vi "LabVIEW_VTOL.vi"() -> ()   [LabVIEW 2018]
uses:
  <vilib>/Analysis/baseanly.llb/A x Vector.vi
  <vilib>/Instr/_visa.llb/VISA Configure Serial Port (Instr).vi
  <vilib>/Analysis/NI_AALBase.lvlib
panel:
  out "Yaw error integral":dbl(graph)
  out "Pitch error intergal":dbl(graph)
  in  "Yaw":dbl(slide) scale=-90.0..90.0
  in  "Pitch":dbl(slide) scale=-90.0..90.0
  out "size(s) 3":i32
  out "size(s) 2":i32
  out "Propeller 2":dbl(graph)
  out "Propeller 1":dbl(graph)
  in  "stop":bool
  out "Raw Data":string
  in  "array type (2D Dbl)":dbl[](array[numeric])
  out "Pitch":T1(graph)
  out "Roll":dbl(graph)
  out "Yaw":T1(graph)
  out "Pitch speed":dbl(graph)
  out "Roll speed":dbl(graph)
  out "Yaw speed":dbl(graph)
  in  "VISA resource name":refnum<visa-resource-name>
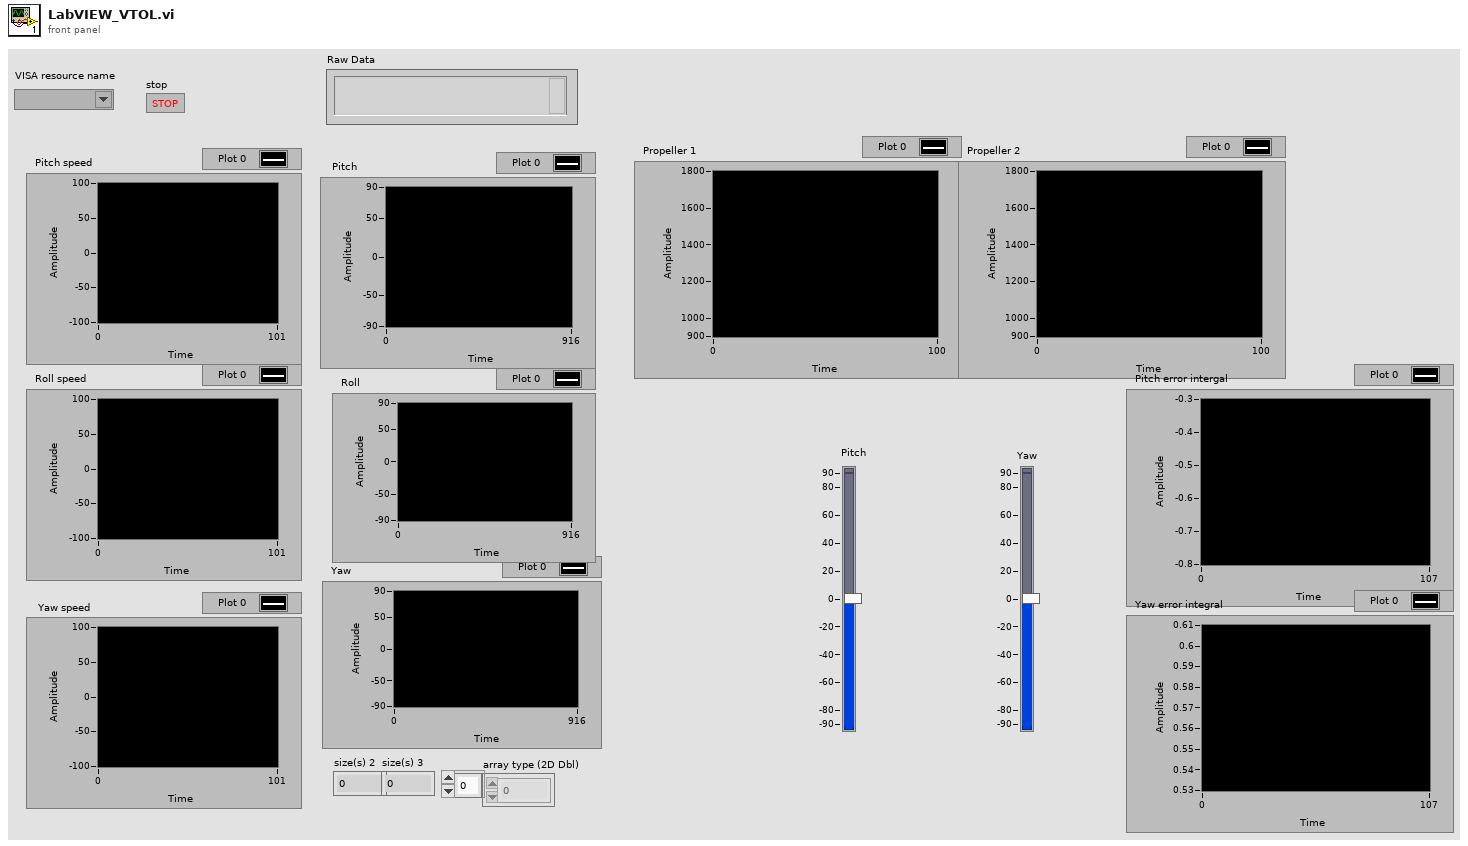
[diagram p1: front panel]
types:
  T1 = cluster{"[0]":dbl, "[1]":dbl, "[2]":dbl, "[3]":dbl, "[4]":dbl, "[5]":dbl, "[6]":dbl, "[7]":dbl, "[8]":dbl}
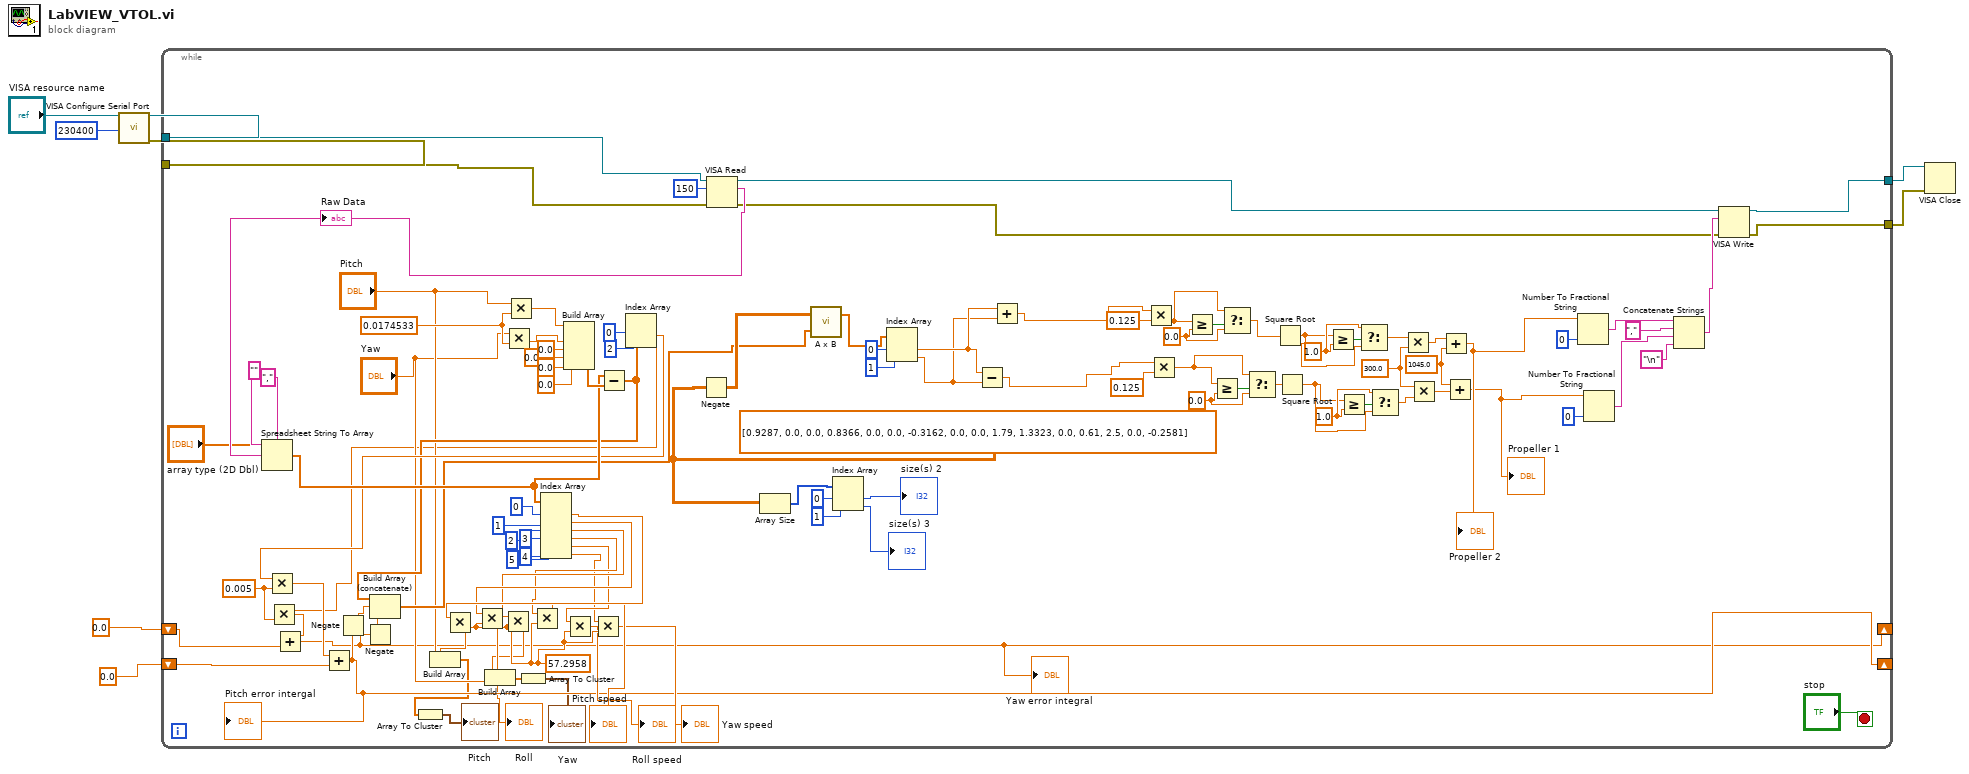
[diagram p0: block diagram]
diagram:
  n1 = call-poly "VISA Configure Serial Port"("VISA resource name"="VISA resource name", "baud rate (9600)"=u32 230400) -> ("VISA resource name out"=w7:refnum<visa-resource-name>, "error out"=w6:errorcluster)  [unwired: 12 in]
  n2 = while {
    tunnel: w7 -> [w113]
    tunnel: w6 -> [w112]
    tunnel: [w59] -> w5
    tunnel: [w56] -> w4
    shift-right: [w29] -> _
    shift-left: 0.0 -> [w14]
    shift-right: [w10] -> _
    shift-left: 0.0 -> [w12]
    stop <- "stop" stop-if-true
    w15 = 0.005 ("y")
    w41 = 0.0174533 ("y")
    w50 = 57.2958 ("y")
    w72 = 1.0 ("y")
    w76 = 1.0 ("y")
    w80 = 0.0 ("y")
    w83 = 0.0 ("y")
    w86 = 1045.0 ("y")
    w89 = 300.0 ("y")
    w9 = dbl[][] [[0.9287, 0.0, 0.0, 0.8366, 0.0, 0.0, -0.3162, 0.0], [0.0, 1.79, 1.3323, 0.0, 0.61, 2.5, 0.0, -0.2581]] ("Controller Gain")
    n3 = Multiply(x="Yaw", y=w41) -> (x*y=w31:dbl)
    n4 = Multiply(x="Pitch", y=w41) -> (x*y=w42:dbl)
    n5 = Build Array(w42, 0.0 ("element"), w31, 0.0 ("element"), 0.0 ("element"), 0.0 ("element")) -> (w37:dbl[])
    n6 = Negate(x=w9) -> (-x=w55:dbl[][])
    n7 = VISA Read(VISA resource name=w113, byte count=u32 150, error in (no error)=w112) -> (VISA resource name out=w58:refnum<visa-resource-name>, read buffer=w110:string, error out=w57:errorcluster)  [unwired: 1 out]
    "Raw Data" <- w110
    n8 = Spreadsheet String To Array(delimiter (Tab)=",", format string="", spreadsheet string=w110, array type (2D Dbl)="array type (2D Dbl)") -> (array=w36:dbl[])
    n9 = Index Array(array=w36, index #1=0 ("index (row)"), index #2=1 ("index (row)"), index #3=2 ("index"), index #4=3 ("index"), index #5=4 ("index"), index #6=5 ("index")) -> (element #1=w52:dbl, element #2=w51:dbl, element #3=w49:dbl, element #4=w48:dbl, element #5=w47:dbl, element #6=w46:dbl)
    n10 = Multiply(x=w52, y=w50) -> (x*y=w27:dbl)
    n11 = Build Array(w27, "Pitch") -> (w22:dbl[])
    n12 = Array To Cluster(array=w22) -> (cluster=→"Pitch":T1)
    n13 = Multiply(x=w51, y=w50) -> (x*y=→"Roll":dbl)
    n14 = Multiply(x=w49, y=w50) -> (x*y=w24:dbl)
    n15 = Build Array(w24, "Yaw") -> (w20:dbl[])
    n16 = Array To Cluster(array=w20) -> (cluster=→"Yaw":T1)
    n17 = Multiply(x=w48, y=w50) -> (x*y=→"Pitch speed":dbl)
    n18 = Multiply(x=w47, y=w50) -> (x*y=→"Roll speed":dbl)
    n19 = Multiply(x=w46, y=w50) -> (x*y=→"Yaw speed":dbl)
    n20 = Subtract(x=w36, y=w37) -> (x-y=w33:dbl[])
    n21 = Index Array(array=w33, index #1=0 ("index"), index #2=2 ("index")) -> (element #1=w34:dbl, element #2=w16:dbl)
    n22 = Multiply(x=w34, y=w15) -> (x*y=w17:dbl)
    n23 = Multiply(x=w16, y=w15) -> (x*y=w13:dbl)
    n24 = Add(x=w13, y=w12) -> (x+y=w10:dbl)
    "Yaw error integral" <- w10
    n25 = Add(x=w17, y=w14) -> (x+y=w29:dbl)
    "Pitch error intergal" <- w29
    n26 = Negate(x=w29) -> (-x=w28:dbl)
    n27 = Negate(x=w10) -> (-x=w11:dbl)
    n28 = Build Array (concatenate)(w33, w28, w11) -> (w32:dbl[])
    n29 = Array Size(array=w9) -> (size(s)=w97:i32[])
    n30 = call-poly <vilib>:"A x B.vi"("Vector"=w32, "A"=w55) -> ("A x Vector"=w94:dbl[])  [unwired: 1 out]
    n31 = Index Array(array=w97, index #1=0 ("index"), index #2=1 ("index")) -> (element #1=→"size(s) 2":i32, element #2=→"size(s) 3":i32)
    n32 = Index Array(array=w94, index #1=0 ("index"), index #2=1 ("index")) -> (element #1=w93:dbl, element #2=w92:dbl)
    n33 = Subtract(x=w93, y=w92) -> (x-y=w53:dbl)
    n34 = Add(x=w93, y=w92) -> (x+y=w54:dbl)
    n35 = Multiply(x=w54, y=0.125) -> (x*y=w84:dbl)
    n36 = Multiply(x=w53, y=0.125) -> (x*y=w78:dbl)
    n37 = Greater Or Equal?(x=w84, y=w83) -> (x >= y?=w85:bool)
    n38 = Greater Or Equal?(x=w78, y=w80) -> (x >= y?=w81:bool)
    n39 = Select(t=w84, s=w85, f=w83) -> (s? t:f=w82:dbl)
    n40 = Select(t=w78, s=w81, f=w80) -> (s? t:f=w79:dbl)
    n41 = Square Root(x=w82) -> (sqrt(x)=w75:dbl)
    n42 = Square Root(x=w79) -> (sqrt(x)=w70:dbl)
    n43 = Greater Or Equal?(x=w75, y=w76) -> (x >= y?=w77:bool)
    n44 = Greater Or Equal?(x=w70, y=w72) -> (x >= y?=w73:bool)
    n45 = Select(t=w76, s=w77, f=w75) -> (s? t:f=w74:dbl)
    n46 = Select(t=w72, s=w73, f=w70) -> (s? t:f=w71:dbl)
    n47 = Multiply(x=w74, y=w89) -> (x*y=w88:dbl)
    n48 = Multiply(x=w89, y=w71) -> (x*y=w87:dbl)
    n49 = Add(x=w88, y=w86) -> (x+y=w61:dbl)
    "Propeller 2" <- w61
    n50 = Add(x=w86, y=w87) -> (x+y=w60:dbl)
    "Propeller 1" <- w60
    n51 = Number To Fractional String(number=w61, precision (6)=i16 0) -> (F-format string=w66:string)  [unwired: 2 in]
    n52 = Number To Fractional String(number=w60, precision (6)=i16 0) -> (F-format string=w64:string)  [unwired: 2 in]
    n53 = Concatenate Strings(w66, "," ("string"), w64, "\n" ("string")) -> (w62:string)
    n54 = VISA Write(VISA resource name=w58, write buffer=w62, error in (no error)=w57) -> (VISA resource name out=w59:refnum<visa-resource-name>, error out=w56:errorcluster)  [unwired: 1 out]
  }
  n55 = VISA Close(VISA resource name=w5, error in (no error)=w4) -> ()  [unwired: 1 out]
